vi "Start SubComponent.vi"(5 "Component ID":u8, 7 "FPGA Interface":refnum<class "FPGA Interface.lvclass">, 8 "error in (no error)":errorcluster, 11 "1553 SubComponent in":refnum<class "1553 SubComponent.lvclass">) -> (0 "error out":errorcluster, 3 "1553 SubComponent out":refnum<class "1553 SubComponent.lvclass">)   [LabVIEW 2020, in "BCI-1553 API.lvlib" / "1553 SubComponent.lvclass"]
doc: "#Virtual\n\nAll children must override this method. Children are expected to provide functionality that 'starts' their operation. This will involve minimal register operations in the 1553 Session component to achieve the fastest possible start.\n\nIdeal Start Order:\n1. Remote Terminals\n2: Bus Monitor\n3. Bus Controller"
uses:
  1553 SubComponent.lvclass
  Dependencies/FPGA Interface/FPGA Interface.lvclass
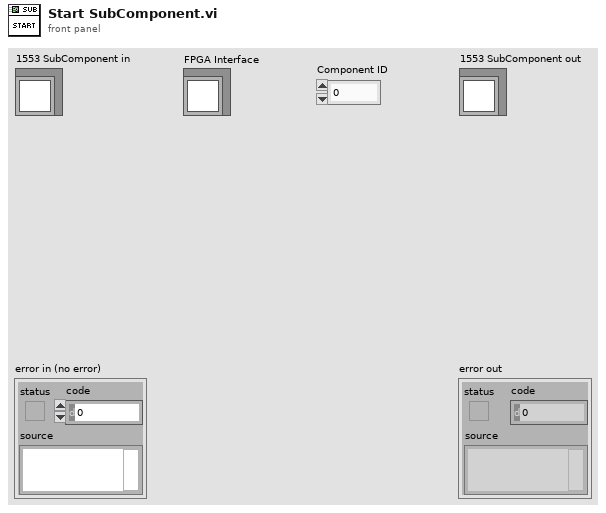
[diagram p1: front panel]
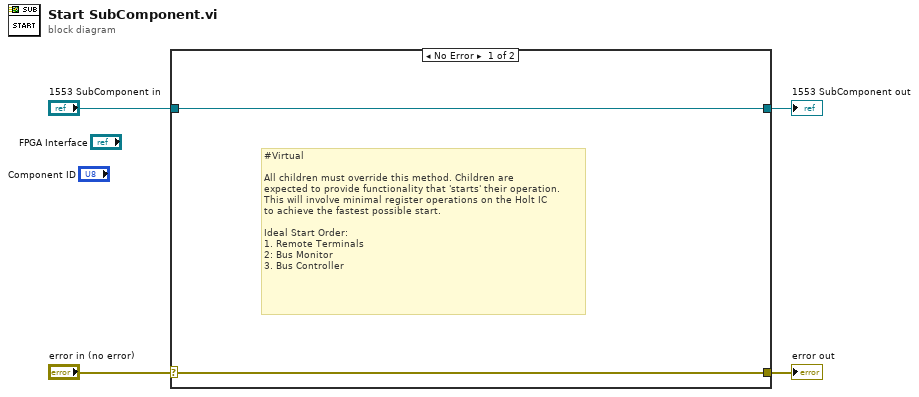
[diagram p0: block diagram]
diagram:
  n1 = case shown="No Error" "error in (no error)" {
    selector: "error in (no error)" -> [w5 w8]
    tunnel: [w5 w8] -> w3
    tunnel: [w6 w7] -> w1
    tunnel: "1553 SubComponent in" -> [w6 w7]
    frame No Error {
      # "#Virtual\n\nAll children must override this method. Children are\nexpected to provide functionality that 'starts' their operation.\nThis will involve minimal register operations on the Holt IC\nto achieve the fastest possible start.\n\nIdeal Start Order:\n1. Remote Terminals\n2: Bus Monitor\n3. Bus Controller"
    }
    frame Error {
    }
  }
  "error out" <- w3
  "1553 SubComponent out" <- w1
